vi "Prototype.vi"(11 "stop":bool) -> (3 "Array":bool[][](array[boolean]))   [LabVIEW 2015]
uses:
  TronVIEWBotAPI/TronVIEWBotAPI.lvlib
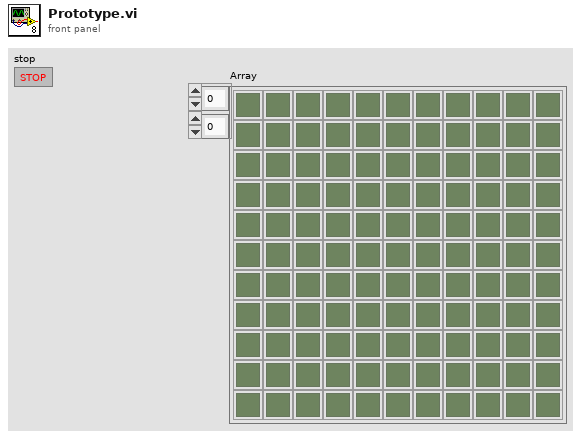
[diagram p1: front panel]
types:
  T1 = typedef "TronVIEWBotAPI.lvlib/MovementDirection.ctl" = enum16{"N", "S", "W", "E"}
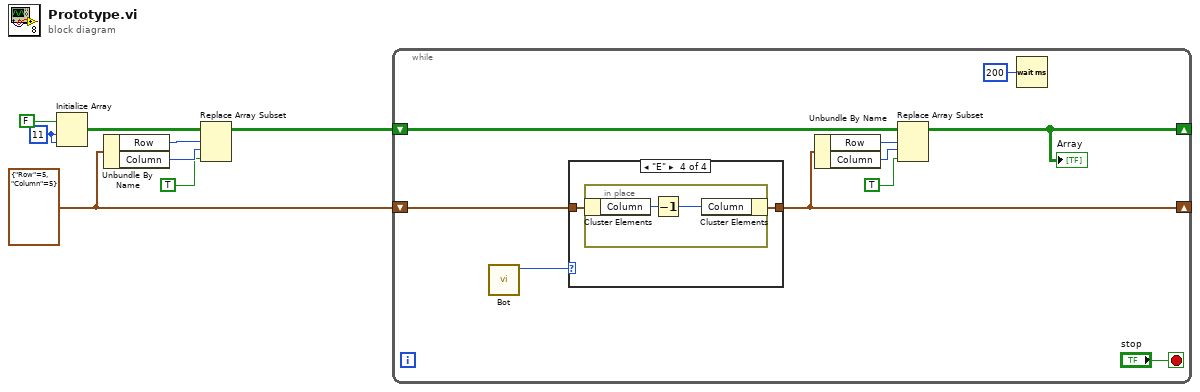
[diagram p0: block diagram]
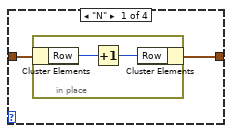
[diagram p2: hidden frame]
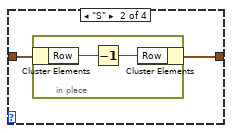
[diagram p3: hidden frame]
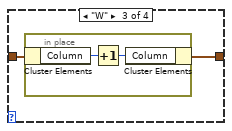
[diagram p4: hidden frame]
diagram:
  w5 = cluster{"Row":i32, "Column":i32} {"Row"=5, "Column"=5}
  w7 = 11 ("dimension size")
  n1 = Initialize Array(FALSE ("Boolean"), w7, w7) -> (w6:bool[][])
  n2 = Unbundle By Name(w5) -> ("Row"=w4:i32, "Column"=w3:i32)
  n3 = Replace Array Subset(array=w6, new element=TRUE ("element"), index (row)=w4, index (col)=w3) -> (w1:bool[][])
  n4 = while {
    shift-right: [w9] -> _
    shift-left: w1 -> [w17]
    shift-right: [w11] -> _
    shift-left: w5 -> [w16]
    stop <- "stop" stop-if-true
    n5 = call "Bot.vi"() -> ("Move"=w15:T1)  [unwired: 10 in, 1 out]
    n6 = case shown="\"E\"" w15 {
      tunnel: w16 -> [w20 w24 w28 w32]
      tunnel: [w19 w23 w27 w31] -> w11
      frame "N" {
        n7 = in-place {
          n8 = in-place-cluster #1(w20) -> ("Row"=w22:i32)
          n9 = Increment(x=w22) -> (x+1=w21:i32)
          n10 = in-place-cluster #1("Row"=w21) -> (w19:cluster{"Row":i32, "Column":i32})
        }
      }
      frame "S" {
        n11 = in-place {
          n12 = in-place-cluster #2(w24) -> ("Row"=w26:i32)
          n13 = Decrement(x=w26) -> (x-1=w25:i32)
          n14 = in-place-cluster #2("Row"=w25) -> (w23:cluster{"Row":i32, "Column":i32})
        }
      }
      frame "W" {
        n15 = in-place {
          n16 = in-place-cluster #3(w28) -> ("Column"=w30:i32)
          n17 = Increment(x=w30) -> (x+1=w29:i32)
          n18 = in-place-cluster #3("Column"=w29) -> (w27:cluster{"Row":i32, "Column":i32})
        }
      }
      frame "E" {
        n19 = in-place {
          n20 = in-place-cluster #4(w32) -> ("Column"=w34:i32)
          n21 = Decrement(x=w34) -> (x-1=w33:i32)
          n22 = in-place-cluster #4("Column"=w33) -> (w31:cluster{"Row":i32, "Column":i32})
        }
      }
    }
    n23 = Unbundle By Name(w11) -> ("Row"=w14:i32, "Column"=w13:i32)
    n24 = Replace Array Subset(array=w17, new element=TRUE ("element"), index (row)=w14, index (col)=w13) -> (w9:bool[][])
    "Array" <- w9
    n25 = Wait (ms)(milliseconds to wait=u32 200) -> ()  [unwired: 1 out]
  }
